vi "resolution.vi"(9 "resolution":dbl) -> (1 "uncertainty":dbl)   [LabVIEW 2021, in "CALIBRATION.lvlib"]
uses:
  CALIBRATION.lvlib
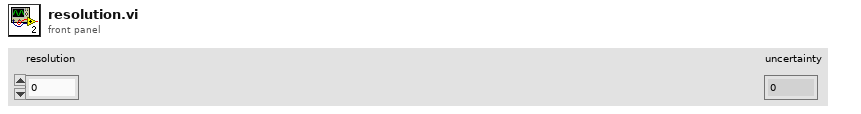
[diagram p1: front panel]
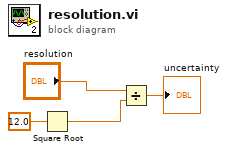
[diagram p0: block diagram]
diagram:
  n1 = Square Root(x=12.0) -> (sqrt(x)=w3:dbl)
  n2 = Divide(x="resolution", y=w3) -> (x/y=→"uncertainty":dbl)
